vi "test_RegisterPinMap_RegisterPinMapFile_PinMapRegistered.vi"(8 "error in":errorcluster) -> (0 "error out":errorcluster, 2 "result":string, 3 "pass":bool)   [LabVIEW 2021, in "MeasurementServerTests.lvlib" / "Pin Map Tests.lvlib"]
uses:
  Pin Map Tests.lvlib
  gRPC/Generated APIs/ni/measurementlink/pinmap/v1/RPC Messages/ni_measurementlink_pinmap_v1_GetPinMapRequest.ctl
  MeasurementServerTests.lvlib
  Runtime/Clients/Pin Map V1/NI Pin Map V1 Client.lvlib
  gRPC/Generated APIs/ni/measurementlink/pinmap/v1/ni.measurementlink.pinmap.v1.api.lvlib
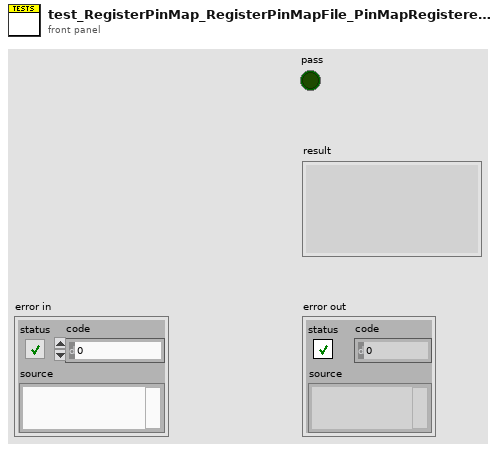
[diagram p1: front panel]
types:
  T1 = typedef "ni.measurementlink.pinmap.v1.api.lvlib/ni_measurementlink_pinmap_v1_GetPinMapRequest.ctl" = cluster{"pin_map_id":string}
  T2 = typedef "grpc-lvsupport-release.lvlib/grpcId.ctl" = u64
  T3 = typedef "ni.measurementlink.pinmap.v1.api.lvlib/ni_measurementlink_pinmap_v1_PinMap.ctl" = cluster{"pin_map_id":string}
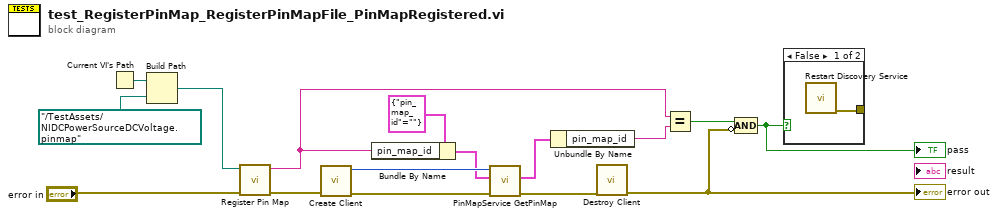
[diagram p0: block diagram]
diagram:
  n1 = Current VI's Path() -> (path=w10:path)
  n2 = Build Path(base path=w10, name or relative path=path "../TestAssets/NIDCPowerSourceDCVoltage.pinmap") -> (appended path=w8:path)
  n3 = call "Register Pin Map.vi"("error in"="error in", "pin map file path"=w8) -> ("error out"=w15:errorcluster, "pin map id"=w1:string)  [unwired: 7 in, 1 out]
  n4 = call "Create Client.vi"("error in"=w15) -> ("error out"=w13:errorcluster, "grpc client id"=w14:T2)  [unwired: 9 in]
  n5 = Bundle By Name(cluster=T1 {"pin_map_id"=""} ("ni_measurementlink_pinmap_v1_GetPinMapRequest"), "pin_map_id"=w1) -> (w3:T1)
  n6 = call "PinMapService GetPinMap.vi"("error in"=w13, "Request Data"=w3, "gRPC ID"=w14) -> ("error out"=w12:errorcluster, "Response Data"=w11:T3)  [unwired: 6 in, 1 out]
  n7 = Unbundle By Name(w11) -> ("pin_map_id"=w7:string)
  n8 = call "Destroy Client.vi"("error in"=w12) -> ("error out"=w6:errorcluster)  [unwired: 10 in]
  "error out" <- w6
  n9 = Equal?(x=w1, y=w7) -> (x = y?=w5:bool)
  n10 = Compound Arithmetic op=AND(w5, invert w6) -> (w4:bool)
  "pass" <- w4
  n11 = case shown="False" w4 {
    tunnel: [w17 _] -> _
    frame False {
      n12 = call "Restart Discovery Service.vi"() -> ("error out"=w17:errorcluster)  [unwired: 11 in]
    }
    frame True {
    }
  }
